vi "Discrete to Continuous.vi"(8 "error in (no error)":errorcluster, 11 "Vessel in":refnum<class "Vessel.lvclass">) -> (0 "error out":errorcluster, 3 "Vessel out":refnum<class "Vessel.lvclass">)   [LabVIEW 2014, in "Vessel.lvclass"]
uses:
  Vessel.lvclass
  Vessel.lvclass/Vessel.ctl
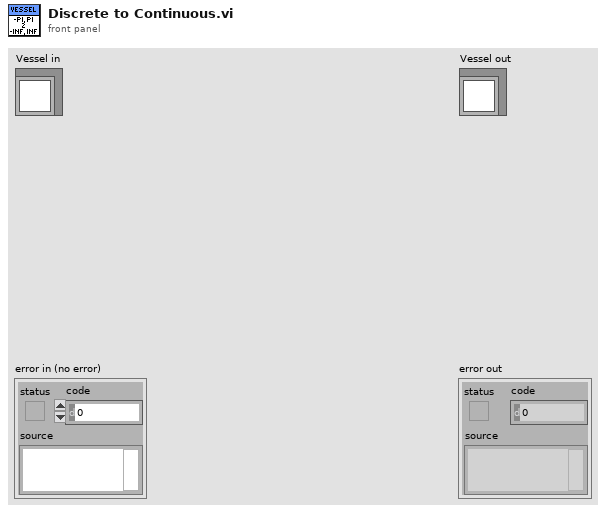
[diagram p1: front panel]
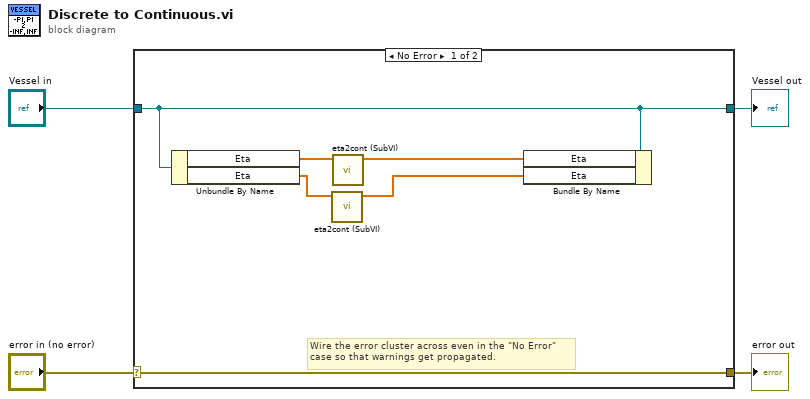
[diagram p0: block diagram]
diagram:
  n1 = case shown="No Error" "error in (no error)" {
    selector: "error in (no error)" -> [w10 w12]
    tunnel: [w10 w12] -> w3
    tunnel: [w8 w11] -> w1
    tunnel: "Vessel in" -> [w8 w11]
    frame No Error {
      # "Wire the error cluster across even in the \"No Error\"\ncase so that warnings get propagated."
      n2 = Unbundle By Name(w8) -> ("Eta"=w9:dbl[], "Eta"=w6:dbl[])
      n3 = call "eta2cont (SubVI).vi"("eta_disc"=w6) -> ("eta_cont"=w5:dbl[])  [unwired: 9 in, 1 out]
      n4 = call "eta2cont (SubVI).vi"("eta_disc"=w9) -> ("eta_cont"=w7:dbl[])  [unwired: 9 in, 1 out]
      n5 = Bundle By Name(cluster=w8, "Eta"=w7, "Eta"=w5) -> ()  [unwired: 1 out]
    }
    frame Error {
    }
  }
  "error out" <- w3
  "Vessel out" <- w1
